vi "HDB3码.vi"() -> ()   [LabVIEW 2013]
panel:
  in  "?":bool
  out "HDB3码波形":i8[](graph)
  out "变换后的HDB3码":i8[](array[numeric])
  in  "输入原消息代码":u32[](array[numeric])
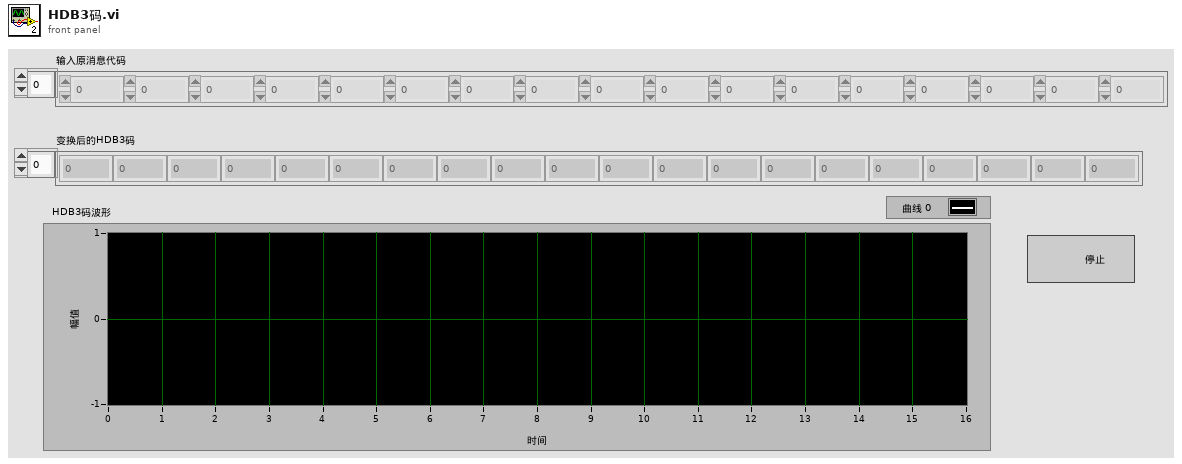
[diagram p1: front panel]
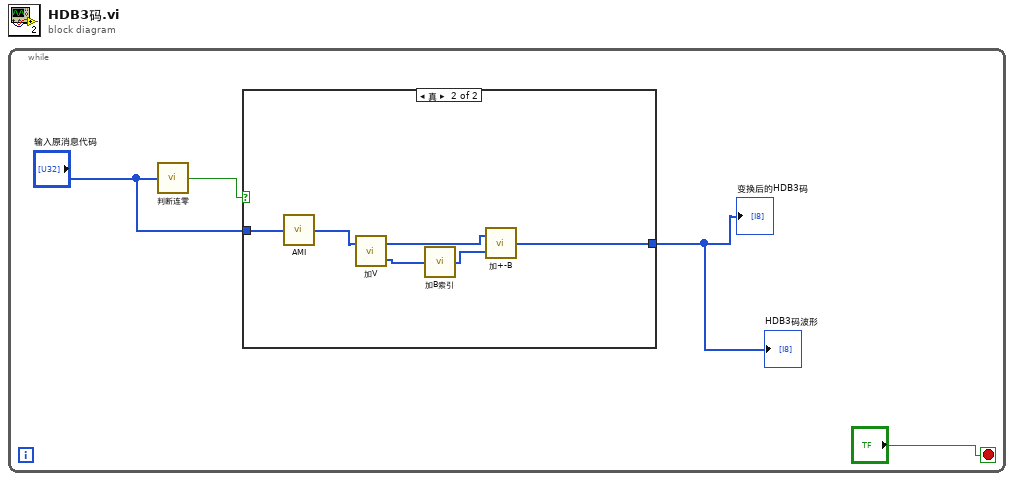
[diagram p0: block diagram]
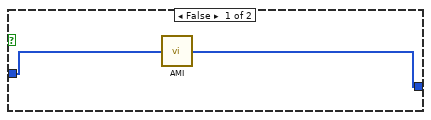
[diagram p2: hidden frame]
diagram:
  n1 = while {
    stop <- "?" stop-if-true
    n2 = call "判断连零.vi"("原消息代码"="输入原消息代码") -> ("布尔"=w4:bool)
    n3 = case shown="真" w4 {
      tunnel: "输入原消息代码" -> [w6 w12]
      tunnel: [w5 w7] -> w2
      frame False {
        n4 = call "AMI.vi"("输入原消息代码"=w6) -> ("变换后的AMI码"=w5:i8[])
      }
      frame True {
        n5 = call "AMI.vi"("输入原消息代码"=w12) -> ("变换后的AMI码"=w11:i8[])
        n6 = call "加V.vi"("接收的AMI码"=w11) -> ("索引值"=w10:u8[], "加+V和-V"=w8:i8[])  [unwired: 1 in]
        n7 = call "加B索引.vi"("索引值"=w10) -> ("加B索引值"=w9:u8[])
        n8 = call "加+-B.vi"("加B索引值"=w9, "加V"=w8) -> ("加B"=w7:i8[])
      }
    }
    "变换后的HDB3码" <- w2
    "HDB3码波形" <- w2
  }
